vi "Time and Proximity Check Data Highway.vi"(8 "error in (no error)":errorcluster, 9 "Time Target (s)":dbl, 10 "Proximity switch":bool, 11 "Timer state variables in":T2) -> (0 "error out":errorcluster, 2 "Status":T1, 3 "Timer state variables out":T2)   [LabVIEW 2012]
uses:
  Type Defs/Timer State Variables.ctl
  Shared Files/Shared Type Defs/Cycle Status Cluster.ctl
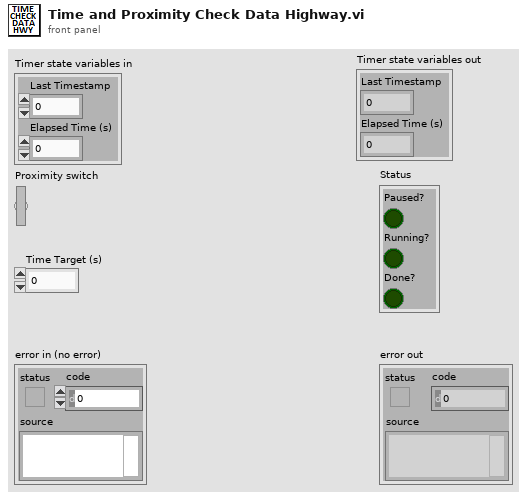
[diagram p1: front panel]
types:
  T1 = typedef "Cycle Status Cluster.ctl" = cluster{"Paused?":bool, "Running?":bool, "Done?":bool}
  T2 = typedef "Timer State Variables.ctl" = cluster{"Last Timestamp":dbl, "Elapsed Time (s)":dbl}
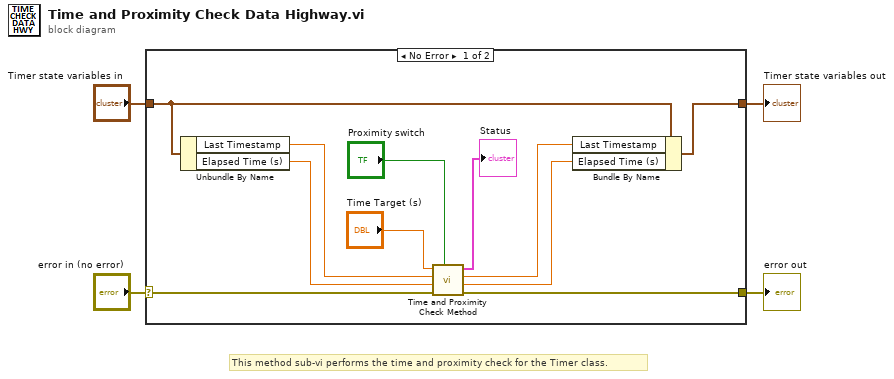
[diagram p0: block diagram]
diagram:
  # "This method sub-vi performs the time and proximity check for the Timer class."
  n1 = case shown="No Error" "error in (no error)" {
    selector: "error in (no error)" -> [w15 w17]
    tunnel: [w14 w17] -> w3
    tunnel: [w10 w16] -> w1
    tunnel: "Timer state variables in" -> [w13 w16]
    frame No Error {
      n2 = Unbundle By Name(w13) -> ("Last Timestamp"=w7:dbl, "Elapsed Time (s)"=w6:dbl)
      n3 = call "Time and Proximity Check Method.vi"("Proximity switch"="Proximity switch", "error in (no error)"=w15, "Elapsed Time (s)"=w6, "Last Time Stamp"=w7, "Time Target (s)"="Time Target (s)") -> ("error out"=w14:errorcluster, "New Elapsed Time (s)"=w8:dbl, "New Time Stamp"=w5:dbl, "Status"=→"Status":T1)  [unwired: 3 in]
      n4 = Bundle By Name(cluster=w13, "Last Timestamp"=w5, "Elapsed Time (s)"=w8) -> (w10:T2)
    }
    frame Error {
    }
  }
  "error out" <- w3
  "Timer state variables out" <- w1
